vi "dfd_Elp Lowpass S Poles and Zeros.vi"(2 "attenuation(dB)":dbl=60.0 format="%.2f", 3 "ripple(dB)":dbl=0.1 format="%.2f", 4 "low cutoff freq: wl":dbl=0.125 format="%.3f", 5 "order":i32=2) -> (0 "zeros":T1[](array[typedef]), 1 "poles":T1[](array[typedef]))   [LabVIEW 2017, in "NI_DigFilter_Design.lvlib"]
uses:
  <vilib>/addons/Digital Filter Design/NI_DigFilter_Design.lvlib
  <vilib>/addons/Digital Filter Design/_Objects.llb/DFD Pole-Zero.ctl
  <vilib>/addons/Digital Filter Design/NI_DigFilterLicensed.lvlib
panel:
  in  "DFD Zero Pole":T1={"value"=0.0+0.0i, "z attr"={"real"=FALSE, "lp"=FALSE, "uc"=FALSE}, "order"=1}
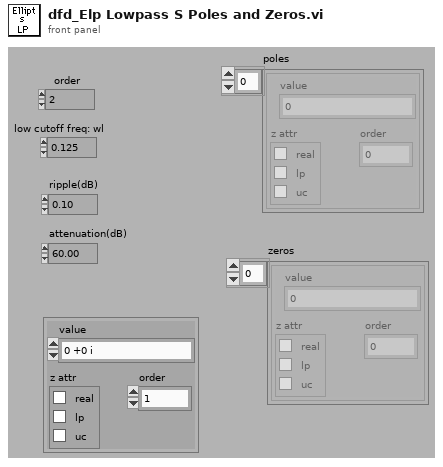
[diagram p1: front panel]
types:
  T1 = typedef "NI_DigFilterLicensed.lvlib/DFD Pole-Zero.ctl" = cluster{"value":cdb, "z attr":cluster{"real":bool, "lp":bool, "uc":bool}, "order":i32}
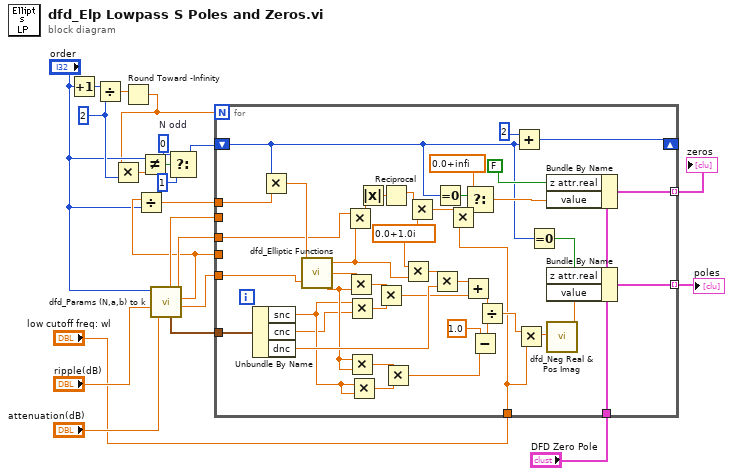
[diagram p0: block diagram]
diagram:
  w10 = 0  # N odd
  w12 = 2
  n1 = Increment(x="order") -> (x+1=w22:i32)
  n2 = Divide(x=w22, y=w12) -> (x/y=w21:dbl)
  n3 = Round Toward -Infinity(1:w21) -> (0:w3:dbl)
  n4 = Multiply(x=w3, y=w12) -> (x*y=w20:dbl)
  n5 = Not Equal?(x="order", y=w20) -> (x != y?=w11:bool)
  n6 = call <vilib>:"dfd_Params (N,a,b) to k.vi"("order"="order", "passband ripple"="ripple(dB)", "stopband attenuation"="attenuation(dB)") -> ("e"=w15:dbl, "Elliptic Primes"=w16:cluster{"snc":dbl, "cnc":dbl, "dnc":dbl}, "k"=w14:dbl, "K"=w7:dbl, "k'"=w13:dbl)  [unwired: 2 out]
  n7 = Divide(x=w7, y="order") -> (x/y=w5:dbl)
  n8 = Select(t=w10, s=w11, f=1) -> (s? t:f=w8:i32)
  n9 = for {
    N: w3 -> [_]
    tunnel: "DFD Zero Pole" -> [w23]
    tunnel: [w65] -> w18 mode=indexing
    tunnel: w16 -> [w63]
    tunnel: w15 -> [_]
    tunnel: w14 -> [w29]
    tunnel: w7 -> [_]
    tunnel: w13 -> [w60]
    shift-right: [w57] -> _
    shift-left: w8 -> [w24]
    tunnel: w5 -> [w62]
    tunnel: [w33] -> w2 mode=indexing
    tunnel: "low cutoff freq: wl" -> [w26]
    w56 = cdb 0.0+1.0i
    n10 = Unbundle By Name(w63) -> ("snc"=w36:dbl, "cnc"=w35:dbl, "dnc"=w46:dbl)
    n11 = Multiply(x=w24, y=w62) -> (x*y=w61:dbl)
    n12 = call <vilib>:"dfd_Elliptic Functions.vi"("u"=w61, "k'"=w60) -> ("sn(k)"=w47:dbl, "cn(k)"=w50:dbl, "dn(k)"=w37:dbl)  [unwired: 1 out]
    n13 = Multiply(x=w29, y=w47) -> (x*y=w54:dbl)
    n14 = Multiply(x=w50, y=w37) -> (x*y=w49:dbl)
    n15 = Multiply(x=w36, y=w35) -> (x*y=w48:dbl)
    n16 = Multiply(x=w37, y=w37) -> (x*y=w39:dbl)
    n17 = Multiply(x=w36, y=w36) -> (x*y=w40:dbl)
    n18 = Absolute Value(x=w54) -> (abs(x)=w59:dbl)
    n19 = Multiply(x=w49, y=w48) -> (x*y=w43:dbl)
    n20 = Reciprocal(x=w59) -> (1/x=w55:dbl)
    n21 = Multiply(x=w39, y=w40) -> (x*y=w38:dbl)
    n22 = Multiply(x=w56, y=w47) -> (x*y=w45:cdb)
    n23 = Multiply(x=w55, y=w56) -> (x*y=w30:cdb)
    n24 = Multiply(x=w45, y=w46) -> (x*y=w44:cdb)
    n25 = Equal To 0?(x=w24) -> (x = 0?=w53:bool)
    n26 = Multiply(x=w30, y=w26) -> (x*y=w28:cdb)
    n27 = Add(x=w44, y=w43) -> (x+y=w42:cdb)
    n28 = Select(t=cdb 0.0+infi, s=w53, f=w28) -> (s? t:f=w51:cdb)
    n29 = Subtract(x=1.0, y=w38) -> (x-y=w34:dbl)
    n30 = Divide(x=w42, y=w34) -> (x/y=w32:cdb)
    n31 = Add(x=2, y=w24) -> (x+y=w57:i32)
    n32 = Multiply(x=w32, y=w26) -> (x*y=w27:cdb)
    n33 = Equal To 0?(x=w24) -> (x = 0?=w25:bool)
    n34 = Bundle By Name(cluster=w23, "z attr.real"=FALSE, "value"=w51) -> (w65:T1)
    n35 = call <vilib>:"dfd_Neg Real & Pos Imag.vi"("complex in"=w27) -> ("complex out"=w31:cdb)
    n36 = Bundle By Name(cluster=w23, "z attr.real"=w25, "value"=w31) -> (w33:T1)
  }
  "poles" <- w2
  "zeros" <- w18
